vi "Go2XYZwWait (SubVI).vi"(0 ".NET Refnum in":refnum<k24>, 5 "Go to Coordinates":T2={"X [mm]"=25.0, "Y [mm]"=12.5, "Z [mm]"=5.0}, 7 "Axis Speeds":T4={"vX [mm/s]"=25.0, "vY [mm/s]"=12.5, "vZ [mm/s]"=5.0}, 11 "error in (no error)":errorcluster) -> (3 "completed":bool, 4 ".NET Refnum out":refnum<k24>, 6 "Final Position":T1, 14 "Initial Position":T3, 15 "error out":errorcluster)   [LabVIEW 2016]
uses:
  C:/Users/Aerotech/Documents/BNLStaveAssembly-blueprint/Bin/Aerotech.A3200.dll
  BNLStaveAssembly-blueprint/Bin/Aerotech.A3200.dll
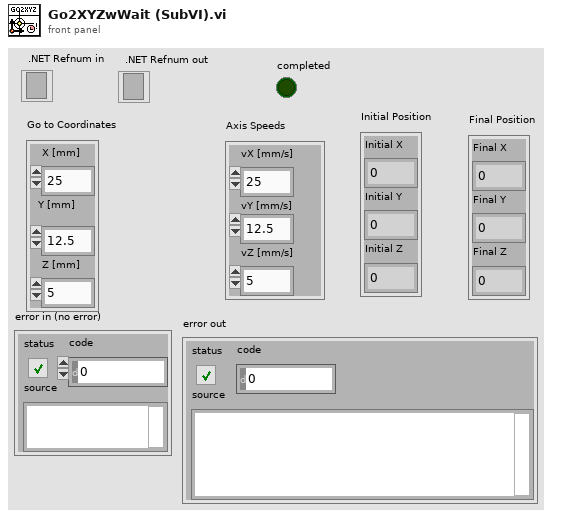
[diagram p1: front panel]
types:
  T1 = cluster{"Final X":dbl, "Final Y":dbl, "Final Z":dbl}
  T2 = cluster{"X [mm]":dbl, "Y [mm]":dbl, "Z [mm]":dbl}
  T3 = cluster{"Initial X":dbl, "Initial Y":dbl, "Initial Z":dbl}
  T4 = cluster{"vX [mm/s]":dbl, "vY [mm/s]":dbl, "vZ [mm/s]":dbl}
  T5 = cluster{"Go to X":dbl, "Go to Y":dbl, "Go to Z":dbl}
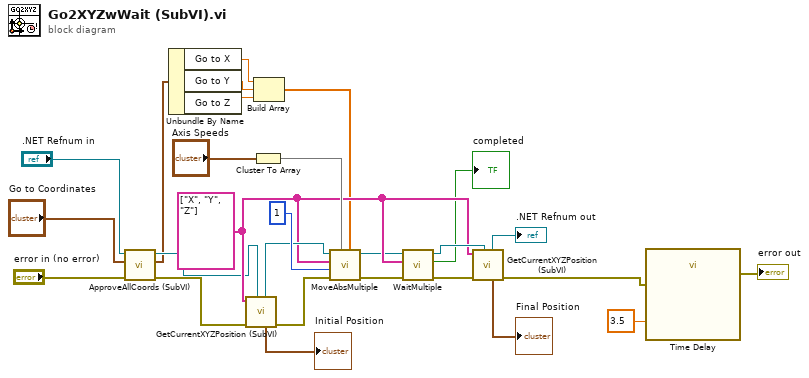
[diagram p0: block diagram]
diagram:
  w19 = string[] ["X", "Y", "Z"]
  n1 = call "ApproveAllCoords (SubVI).vi"("error in (no error)"="error in (no error)", "Go to Coordinates"="Go to Coordinates", "Controller .NET Refnum in"=".NET Refnum in") -> ("error out"=w17:errorcluster, "Approved Coordinates"=w12:T5, "Controller .NET Refnum out"=w13:refnum<k24>)  [unwired: 6 in]
  n2 = Unbundle By Name(w12) -> ("Go to X"=w14:dbl, "Go to Y"=w15:dbl, "Go to Z"=w16:dbl)
  n3 = call "GetCurrentXYZPosition (SubVI).vi"(".NET Refnum in - Device"=w13, "error in (no error)"=w17, "Axes Names"=w19) -> ("error out"=w26:errorcluster, "Current stage position"=→"Initial Position":T2, ".NET Refnum out  - Device"=w25:refnum<k24>)  [unwired: 3 in, 3 out]
  n4 = Cluster To Array(cluster="Axis Speeds") -> (array=w23:dbl[])
  n5 = Build Array(w14, w15, w16) -> (w9:dbl[])
  n6 = call "MoveAbsMultiple.vi"("positions"=w9, "speeds"=w23, "error in (no error)"=w26, "taskId"=1 ("taskNumber"), "axis names"=w19, "controller in"=w25) -> ("error out"=w8:errorcluster, "controller out"=w7:refnum<k24>)  [unwired: 4 in]
  n7 = call "WaitMultiple.vi"("error in (no error)"=w8, "axis names"=w19, "controller in"=w7) -> ("error out"=w20:errorcluster, "completed"=→"completed":bool, "controller out"=w22:refnum<k24>)  [unwired: 6 in]
  n8 = call "GetCurrentXYZPosition (SubVI).vi"(".NET Refnum in - Device"=w22, "error in (no error)"=w20, "Axes Names"=w19) -> ("error out"=w3:errorcluster, "Current stage position"=→"Final Position":T2, ".NET Refnum out  - Device"=→".NET Refnum out":refnum<k24>)  [unwired: 3 in, 3 out]
  n9 = call "Time Delay"("error in (no error)"=w3, "Delay Time (s)"=3.5) -> ("error out"=→"error out":errorcluster)  [unwired: 9 in]
